vi "4155C Take Sample v3.0.vi"(0 "VISA resource name in":refnum<visa-resource-name>, 1 "Emergency Stop":refnum<vi>, 2 "Sample - Gate":u32(ring)=2 items=["SMU1  ", "SMU2  ", "SMU3  ", "SMU4  ", "SMU5  ", "SMU6  ", "VSU1  ", "VSU2  "], 5 "Vg":dbl min=-100.0 max=100.0 format="%.2f", 7 "Sample - Drain":u32(ring)=1 items=["SMU1  ", "SMU2  ", "SMU3  ", "SMU4  ", "SMU5  ", "SMU6  ", "VSU1  ", "VSU2  "], 9 "Vd":dbl min=-100.0 max=100.0 format="%.2f", 11 "error in (no error)":errorcluster) -> (3 "Time":dbl[](array[numeric]) format="%.2f", 4 "VISA Resource Name out":refnum<visa-resource-name>, 6 "Ig":dbl[](array[numeric]) format="%.2f", 10 "Id":dbl[](array[numeric]) format="%.2f", 14 "Is":dbl[](array[numeric]) format="%.2f", 15 "error out":errorcluster)   [LabVIEW 2016]
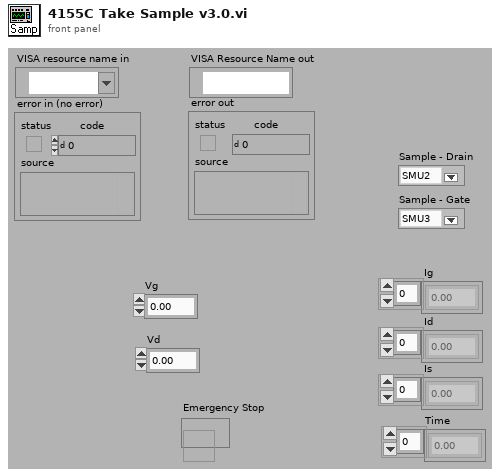
[diagram p1: front panel]
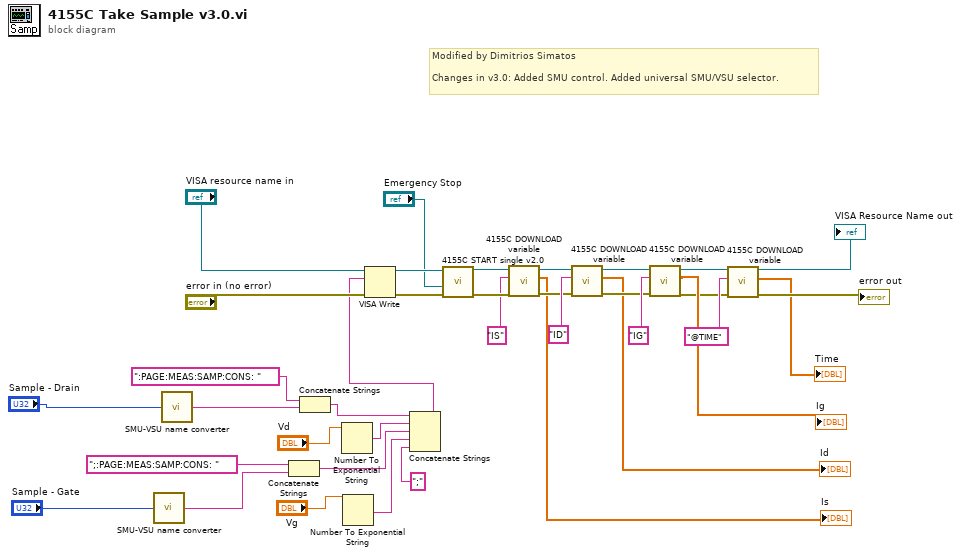
[diagram p0: block diagram]
diagram:
  # "Modified by Dimitrios Simatos\n\nChanges in v3.0: Added SMU control. Added universal SMU/VSU selector."
  n1 = call "SMU-VSU name converter.vi"("unit to configure"="Sample - Gate") -> ("SMU/VSU to be configured"=w1:string)
  n2 = call "SMU-VSU name converter.vi"("unit to configure"="Sample - Drain") -> ("SMU/VSU to be configured"=w5:string)
  n3 = Concatenate Strings(";:PAGE:MEAS:SAMP:CONS: " ("write buffer (\"\")"), w1) -> (w3:string)
  n4 = Concatenate Strings(":PAGE:MEAS:SAMP:CONS: " ("write buffer (\"\")"), w5) -> (w8:string)
  n5 = Number To Exponential String(number="Vd") -> (E-format string=w36:string)  [unwired: 3 in]
  n6 = Number To Exponential String(number="Vg") -> (E-format string=w34:string)  [unwired: 3 in]
  n7 = Concatenate Strings(w8, w36, w3, w34, ";" ("Substring")) -> (w31:string)
  n8 = VISA Write(VISA resource name="VISA resource name in", write buffer=w31, error in (no error)="error in (no error)") -> (VISA resource name out=w30:refnum<visa-resource-name>, error out=w29:errorcluster)  [unwired: 1 out]
  n9 = call "4155C START single v2.0.vi"("error in (no error)"=w29, "Emergency Stop"="Emergency Stop", "VISA resource name in"=w30) -> ("error out"=w26:errorcluster, "VISA Resource Name out"=w27:refnum<visa-resource-name>)  [unwired: 3 in]
  n10 = call "4155C DOWNLOAD variable.vi"("error in (no error)"=w26, "Variable name"="IS", "VISA resource name in"=w27) -> ("error out"=w23:errorcluster, "Output data"=→"Is":dbl[], "VISA Resource Name out"=w22:refnum<visa-resource-name>)  [unwired: 2 in]
  n11 = call "4155C DOWNLOAD variable.vi"("error in (no error)"=w23, "Variable name"="ID", "VISA resource name in"=w22) -> ("error out"=w20:errorcluster, "Output data"=→"Id":dbl[], "VISA Resource Name out"=w19:refnum<visa-resource-name>)  [unwired: 2 in]
  n12 = call "4155C DOWNLOAD variable.vi"("error in (no error)"=w20, "Variable name"="IG", "VISA resource name in"=w19) -> ("error out"=w12:errorcluster, "Output data"=→"Ig":dbl[], "VISA Resource Name out"=w13:refnum<visa-resource-name>)  [unwired: 2 in]
  n13 = call "4155C DOWNLOAD variable.vi"("error in (no error)"=w12, "Variable name"="@TIME", "VISA resource name in"=w13) -> ("error out"=→"error out":errorcluster, "Output data"=→"Time":dbl[], "VISA Resource Name out"=→"VISA Resource Name out":refnum<visa-resource-name>)  [unwired: 2 in]
